vi "Демультиплексор.vi"(2 "?":bool, 3 "?":bool) -> (0 "2":bool, 1 "1":bool)   [LabVIEW 2012]
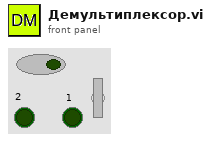
[diagram p1: front panel]
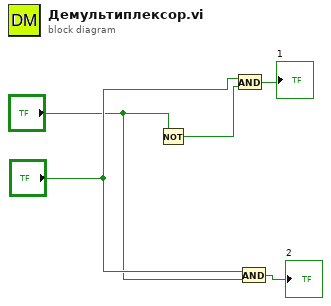
[diagram p0: block diagram]
diagram:
  n1 = Not(x="?") -> (.not. x?=w4:bool)
  n2 = And(x="?", y=w4) -> (x .and. y?=→"1":bool)
  n3 = And(x="?", y="?") -> (x .and. y?=→"2":bool)
